vi "UART.vi"() -> ()   [LabVIEW 2014]
uses:
  <vilib>/MakerHub/LINX/Public/Utilities/Open Local.vi
  <vilib>/Instr/_visa.llb/VISA Configure Serial Port (Instr).vi
  <vilib>/MakerHub/LINX/LMH-LINX.lvlib
panel:
  out "Result Event 2":bool
  out "Result Event":bool
  in  "Event":bool
  in  "stop 2":bool
  out "resulting string":string
  in  "index":i32
  out "find list":string[](array[string])
  out "Error Out":errorcluster
  out "Data":string
  out "Bytes Available":u8
  out "Numeric":i32
  in  "stop":bool
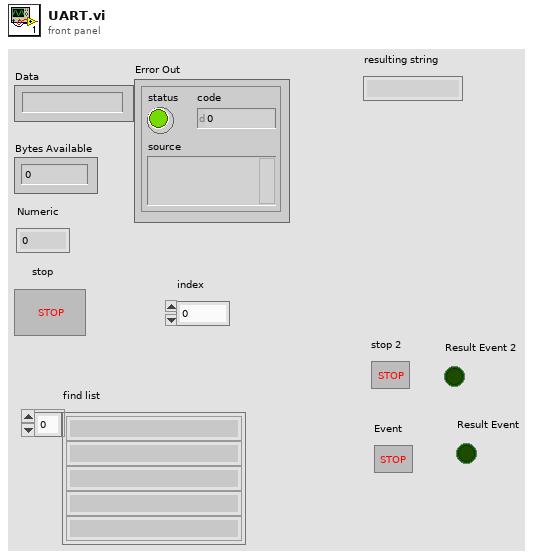
[diagram p1: front panel]
types:
  T1 = enum16{"init", "Write", "CheckData", "Read", "Delay", "Stop"}
  T2 = typedef "LMH-LINX.lvlib/LINX Ref.ctl" = cluster{"IO":T3, "Interface":T4, "LINX Device Config":T5}
  T3 = typedef "LMH-LINX.lvlib/Platform.ctl" = enum16{"Remote", "Local"}
  T4 = typedef "LMH-LINX.lvlib/Interface.ctl" = enum16{"Serial", "TCP"}
  T5 = typedef "LMH-LINX.lvlib/Device.lvlib/LINX Device Config.ctl" = cluster{"Interface":T4, "COM Port":refnum<visa-resource-name>, "TCP Configuration":T6, "Device Family":u8, "Device ID":u8, "Device Name":string, "TCP Ref":refnum<k5>, "Channels":T7}
  T6 = typedef "LMH-LINX.lvlib/Device.lvlib/TCP Config.ctl" = cluster{"IP Address":string, "Port":u16}
  T7 = typedef "LMH-LINX.lvlib/Channels.ctl" = cluster{"DI":u8[], "DO":u8[], "AI":u8[], "AO":u8[], "PWM":u8[], "QE":u8[], "UART":u8[], "I2C 2":u8[], "SPI":u8[], "CAN":u8[], "Servo":u8[], "AI Ref (V)":dbl, "AI Resolution (Bits)":u8, "AO Ref (V)":dbl, "AO Resolution (Bits)":u8}
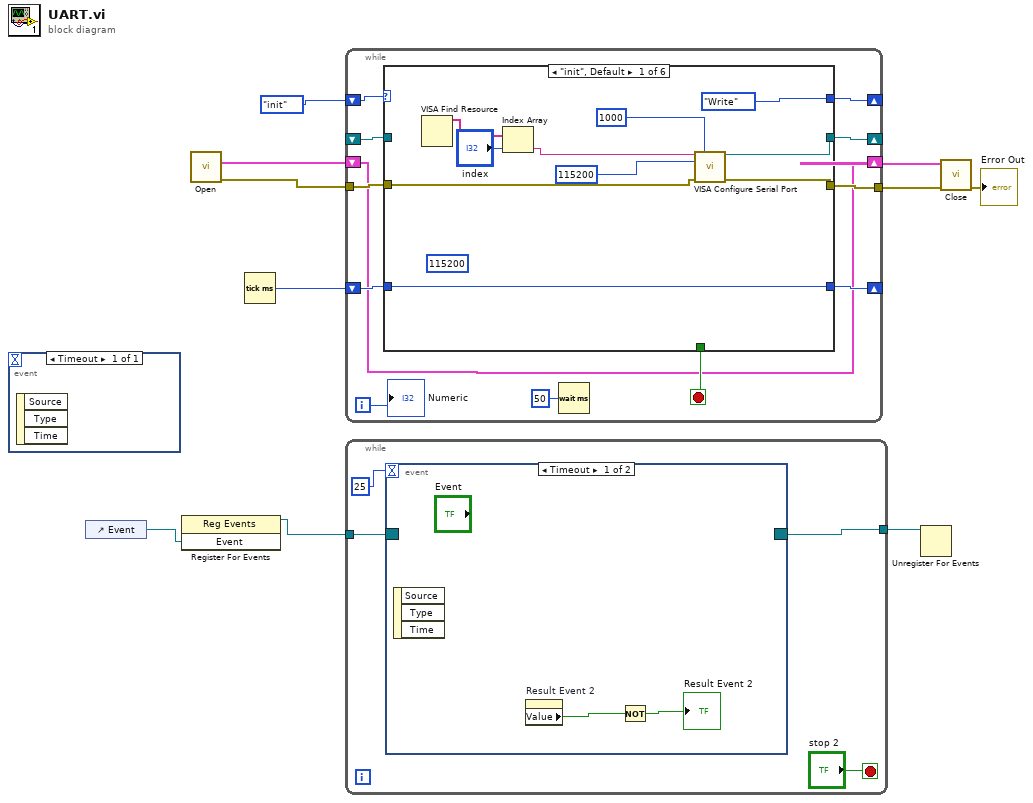
[diagram p0: block diagram]
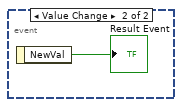
[diagram p2: hidden frame]
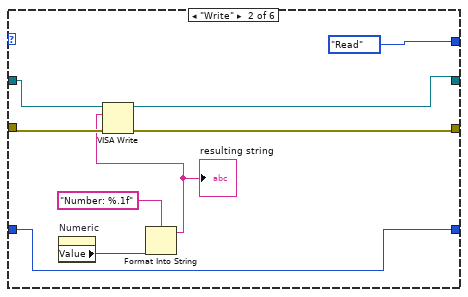
[diagram p3: hidden frame]
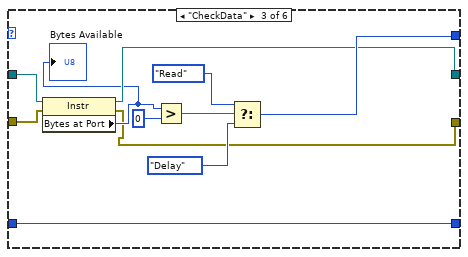
[diagram p4: hidden frame]
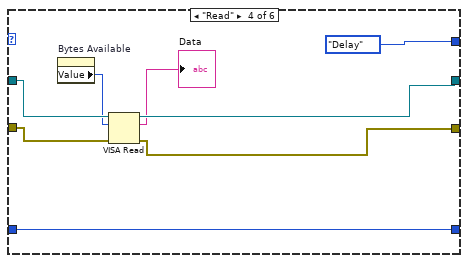
[diagram p5: hidden frame]
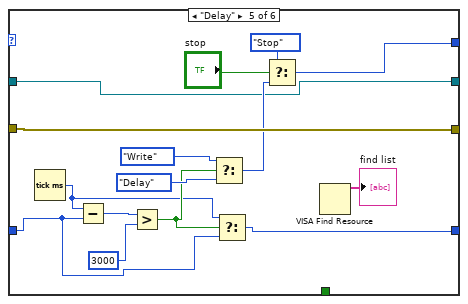
[diagram p6: hidden frame]
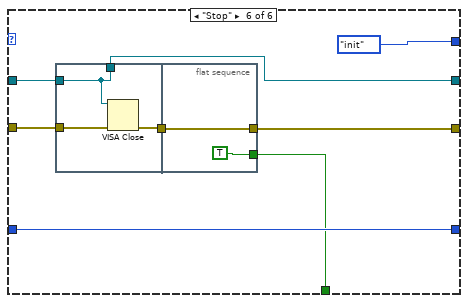
[diagram p7: hidden frame]
diagram:
  n1 = event shown="[0] Timeout" {
    selector: _ -> [_]
    dyn-events: _ -> [_]
    timeout: _ -> [_]
    event Timeout {
      n2 = event-data() -> ()  [unwired: 1 in, 3 out]
    }
  }
  n3 = control-ref of="Event"() -> (w1:refnum<vi>)
  n4 = register-events(w1) -> (reference out=w3:refnum<event-registration>)  [unwired: 2 in, 1 out]
  n5 = call-poly <vilib>:"Open.vi"() -> ("Error Out"=w8:errorcluster, "LINX Resource"=w9:T2)  [unwired: 9 in, 1 out]
  n6 = Tick Count (ms)() -> (millisecond timer value=w5:u32)
  n7 = while {
    tunnel: w8 -> [w22]
    shift-right: [w12] -> w7
    shift-left: w9 -> [w12]
    tunnel: [w20] -> w6
    shift-right: [w14] -> _
    shift-left: T1."init" -> [w21]
    shift-right: [w17] -> _
    shift-left: w5 -> [w16]
    shift-right: [w13] -> _
    shift-left: _ -> [w11]
    i -> [w19]
    stop <- w18 stop-if-true
    n8 = case shown="\"init\", Default" w21 {
      tunnel: w22 -> [w28 w35 w45 w55 w75 w83]
      tunnel: [w29 w34 w42 w56 w75 w78] -> w20
      tunnel: [T1."Write" T1."Read" w48 T1."Delay" w72 T1."init" ("t")] -> w14
      tunnel: [_ _ _ _ _ w79] -> w18
      tunnel: [w31 w38 w47 w59 w63 w81] -> w17
      tunnel: w16 -> [w31 w38 w47 w59 w64 w81]
      tunnel: [w30 w36 w44 w57 w61 w76] -> w13
      tunnel: w11 -> [_ w37 w46 w58 w61 w77]
      frame "init", Default {
        (unwired) u32 115200 ("Baud Rate (9600)")
        n9 = VISA Find Resource() -> (3:w27:string[])  [unwired: 3 in, 2 out]
        n10 = Index Array(array=w27, index="index") -> (element=w25:string)
        n11 = call-poly "VISA Configure Serial Port"("VISA resource name"=w25, "timeout (10sec)"=u32 1000, "baud rate (9600)"=u32 115200, "error in (no error)"=w28) -> ("VISA resource name out"=w30:refnum<visa-resource-name>, "error out"=w29:errorcluster)  [unwired: 10 in]
      }
      frame "Write" {
        n12 = property on="Numeric" class="DigNum (strict)"() -> ("Value"=w40:i32)  [unwired: 2 in, 2 out]
        n13 = Format Into String(format string="Number: %.1f", w40) -> (resulting string=w33:string)  [unwired: 2 in, 1 out]
        "resulting string" <- w33
        n14 = VISA Write(VISA resource name=w37, write buffer=w33, error in (no error)=w35) -> (VISA resource name out=w36:refnum<visa-resource-name>, error out=w34:errorcluster)  [unwired: 1 out]
      }
      frame "CheckData" {
        n15 = property class="Instr"(reference=w46, error in=w45) -> (reference out=w44:refnum<visa-resource-name>, error out=w42:errorcluster, "Bytes at Port"=w43:u32)
        "Bytes Available" <- w43
        n16 = Greater?(x=w43, y=u8 0) -> (0:w51:bool)
        n17 = Select(t=T1."Read", s=w51, f=T1."Delay") -> (s? t:f=w48:T1)
      }
      frame "Read" {
        n18 = property on="Bytes Available" class="DigNum (strict)"() -> ("Value"=w54:u8)  [unwired: 2 in, 2 out]
        n19 = VISA Read(VISA resource name=w58, byte count=w54, error in (no error)=w55) -> (VISA resource name out=w57:refnum<visa-resource-name>, read buffer=→"Data":string, error out=w56:errorcluster)  [unwired: 1 out]
      }
      frame "Delay" {
        n20 = Tick Count (ms)() -> (millisecond timer value=w65:u32)
        n21 = Subtract(x=w65, y=w64) -> (x-y=w71:u32)
        n22 = Greater?(x=w71, y=3000) -> (0:w66:bool)
        n23 = Select(t=T1."Write", s=w66, f=T1."Delay") -> (s? t:f=w67:T1)
        n24 = Select(t=w65, s=w66, f=w64) -> (s? t:f=w63:u32)
        n25 = Select(t=T1."Stop", s="stop", f=w67) -> (s? t:f=w72:T1)
        n26 = VISA Find Resource() -> (3:→"find list":string[])  [unwired: 3 in, 2 out]
      }
      frame "Stop" {
        n27 = flat-sequence {
          tunnel: w83 -> [w86]
          tunnel: [w85] -> w80
          tunnel: w77 -> [w84]
          tunnel: [w84] -> w76
          tunnel: [w88] -> w78
          tunnel: w80 -> [w88]
          tunnel: [TRUE] -> w79
          frame #0 {
            n28 = VISA Close(VISA resource name=w84, error in (no error)=w86) -> (error out=w85:errorcluster)
          }
          frame #1 {
          }
        }
      }
    }
    n29 = Wait (ms)(milliseconds to wait=u32 50) -> ()  [unwired: 1 out]
    "Numeric" <- w19
  }
  n30 = while {
    tunnel: w3 -> [w90]
    tunnel: [w89] -> w2
    stop <- "stop 2" stop-if-true
    n31 = event shown="[0] Timeout" {
      selector: w90 -> [_ _]
      dyn-events: [_ _] -> w89
      timeout: 25 -> [_ _]
      event Timeout {
        n32 = event-data() -> ()  [unwired: 1 in, 3 out]
        n33 = property on="Result Event 2" class="Bool (strict)"() -> ("Value"=w93:bool)  [unwired: 2 in, 2 out]
        n34 = Not(x=w93) -> (.not. x?=→"Result Event 2":bool)
      }
      event Value Change {
        n35 = event-data() -> ("NewVal"=→"Result Event":bool)  [unwired: 1 in]
      }
    }
  }
  n36 = Unregister For Events(event registration refnum=w2) -> ()  [unwired: 1 in, 1 out]
  n37 = call <vilib>:"Close.vi"("Error In"=w6, "LINX Resource"=w7) -> ("Error Out"=→"Error Out":errorcluster)  [unwired: 9 in]
